vi "HEWH Cut Out Flag.vi"(8 "Error In":errorcluster) -> (0 "Error Out":errorcluster)   [LabVIEW 2016]
uses:
  Utility/Type Definitions/UTILITY Notifier.ctl
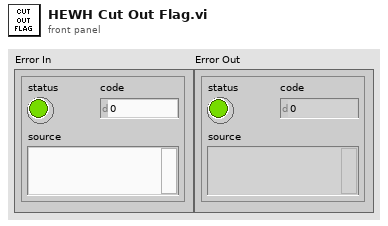
[diagram p1: front panel]
types:
  T1 = typedef "UTILITY Notifier.ctl" = enum16{"Set", "Read", "Release Ref"}
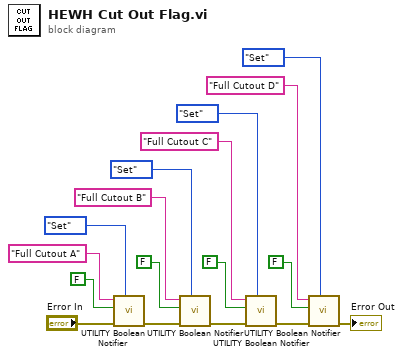
[diagram p0: block diagram]
diagram:
  n1 = call "UTILITY Boolean Notifier.vi"("Status"=UTILITY_Notifier."Set", "error in (no error)"="Error In", "Set Status"=FALSE, "name (unnamed)"="Full Cutout A") -> ("error out"=w5:errorcluster)  [unwired: 6 in, 1 out]
  n2 = call "UTILITY Boolean Notifier.vi"("Status"=UTILITY_Notifier."Set", "error in (no error)"=w5, "Set Status"=FALSE, "name (unnamed)"="Full Cutout B") -> ("error out"=w4:errorcluster)  [unwired: 6 in, 1 out]
  n3 = call "UTILITY Boolean Notifier.vi"("Status"=UTILITY_Notifier."Set", "error in (no error)"=w4, "Set Status"=FALSE, "name (unnamed)"="Full Cutout C") -> ("error out"=w3:errorcluster)  [unwired: 6 in, 1 out]
  n4 = call "UTILITY Boolean Notifier.vi"("Status"=UTILITY_Notifier."Set", "error in (no error)"=w3, "Set Status"=FALSE, "name (unnamed)"="Full Cutout D") -> ("error out"=→"Error Out":errorcluster)  [unwired: 6 in, 1 out]
